vi "NTV_AutoStepcolor.vi"(7 "Read(f) Write(t)":bool, 11 "Color":u32(colorbox)) -> (3 "Color 2":u32(colorbox))   [LabVIEW 2020]
uses:
  <vilib>/Rock Robotics/Network Tables/NT Read Integer.vi
  <vilib>/Rock Robotics/Network Tables/NT Write Integer.vi
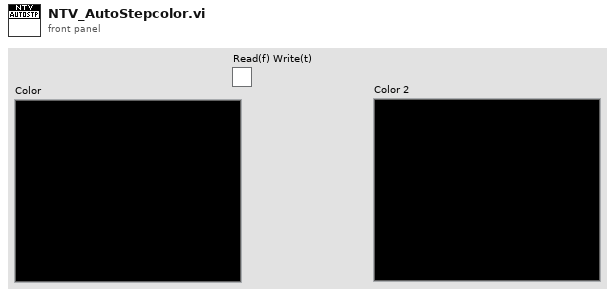
[diagram p1: front panel]
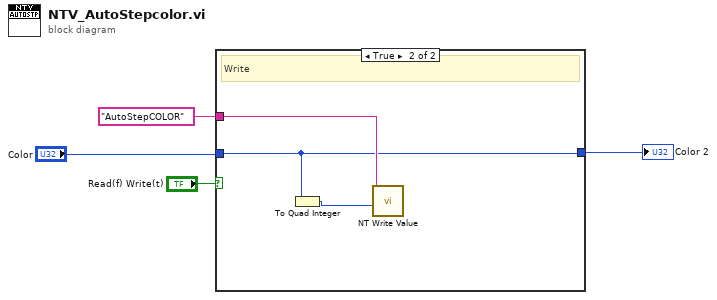
[diagram p0: block diagram]
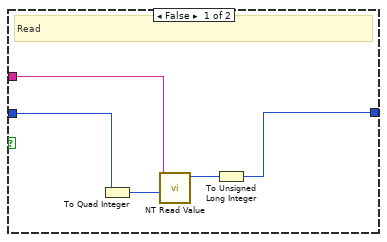
[diagram p2: hidden frame]
diagram:
  n1 = case shown="True" "Read(f) Write(t)" {
    tunnel: "Color" -> [w7 w10]
    tunnel: "AutoStepCOLOR" ("Name") -> [w9 w12]
    tunnel: [w5 w10] -> w1
    frame False {
      # "Read"
      n2 = To Quad Integer(1:w7) -> (0:w8:i64)
      n3 = call-poly <vilib>:"NT Read Value.vi"("default value"=w8, "name"=w9) -> ("value"=w6:i64)  [unwired: 7 in, 2 out]
      n4 = To Unsigned Long Integer(number=w6) -> (unsigned 32bit integer=w5:u32)
    }
    frame True {
      # "Write"
      n5 = To Quad Integer(1:w10) -> (0:w11:i64)
      n6 = call-poly <vilib>:"NT Write Value.vi"("value"=w11, "name"=w12) -> ()  [unwired: 9 in, 1 out]
    }
  }
  "Color 2" <- w1
